vi "Queue Receive.vi"(11 "Queue Actor in":refnum<class "Queue Actor.lvclass">) -> (2 "Msg":refnum<class "Msg.lvclass">, 3 "Queue Actor out":refnum<class "Queue Actor.lvclass">)   [LabVIEW 2021, in "jettl.lvlib" / "Queue Actor.lvclass"]
uses:
  Queue Actor.lvclass
  Msg/Msg/Msg.lvclass
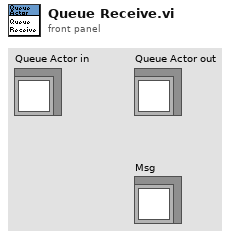
[diagram p1: front panel]
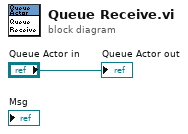
[diagram p0: block diagram]
diagram:
  "Queue Actor out" <- "Queue Actor in"
